vi "getDeviceType.vi"(8 "error in":errorcluster, 11 "connection ID":i32) -> (0 "error out":errorcluster, 2 "devicetype":string, 3 "connection ID":i32)   [LabVIEW 2016]
doc: "This function gets the device type based on its EEPROM configuration."
panel:
  out "params_cluster":cluster{"Numeric":i32}
  in  "Params_cluster":cluster{"Numeric":dbl}
  in  "results_cluster":cluster{"errNo":i32, "devicetype":string}
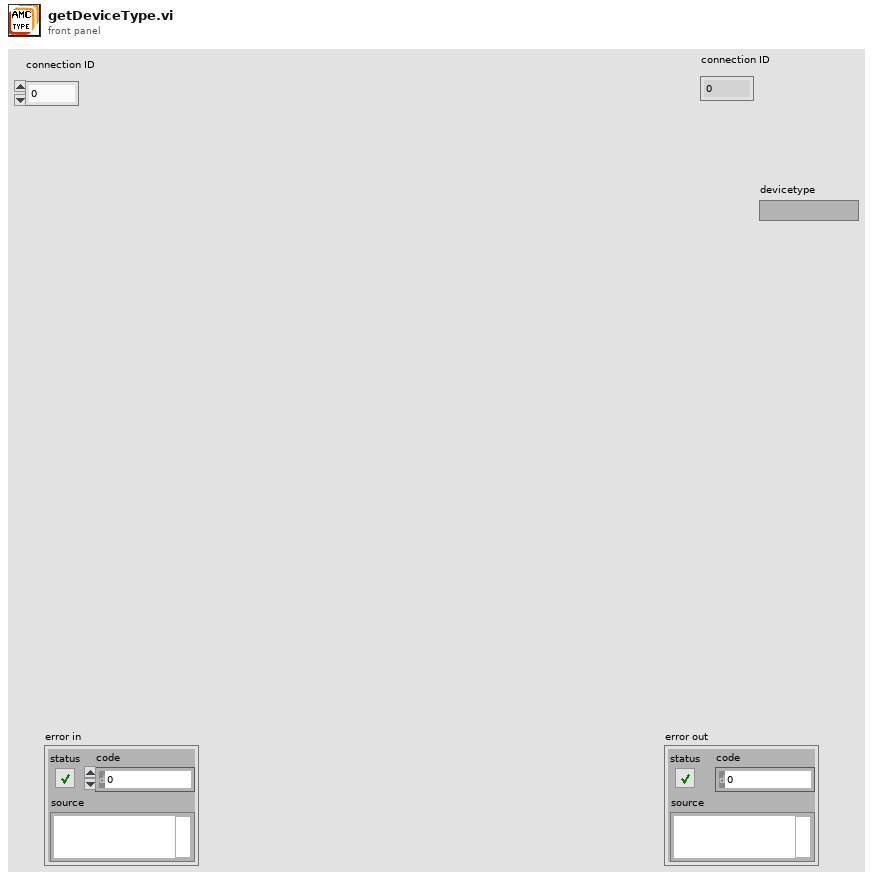
[diagram p1: front panel]
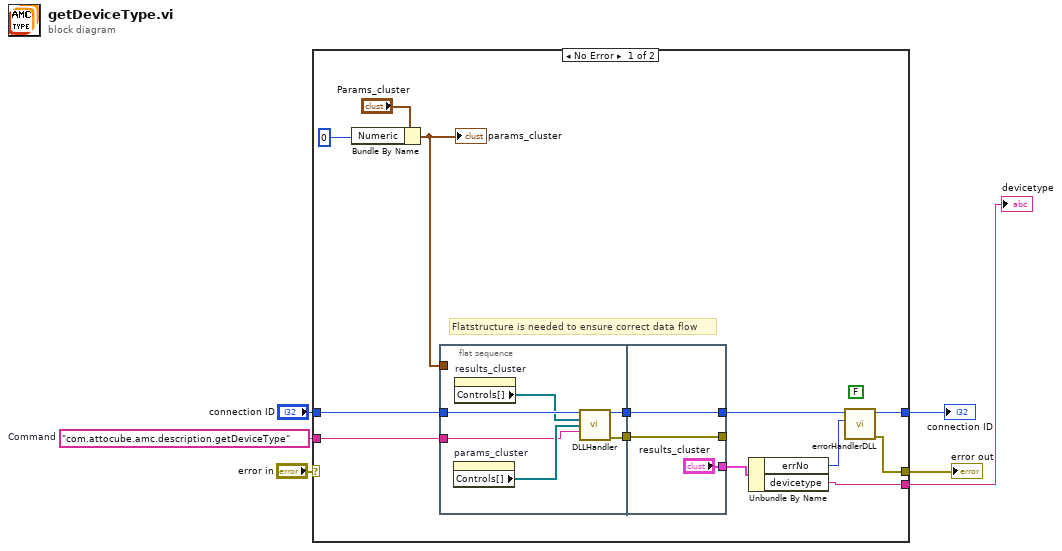
[diagram p0: block diagram]
diagram:
  w4 = "com.attocube.amc.description.getDeviceType"  # Command
  n1 = case shown="No Error" "error in" {
    selector: "error in" -> [_ w30]
    tunnel: [w9 w30] -> w6
    tunnel: "connection ID" -> [w19 w29]
    tunnel: w4 -> [w16 _]
    tunnel: [w11 w29] -> w2
    tunnel: [w7 _] -> w1
    frame No Error {
      (unwired) FALSE ("show popup")
      # "Flatstructure is needed to ensure correct data flow"
      n2 = Bundle By Name(cluster="Params_cluster", "Numeric"=0) -> (w14:cluster{"Numeric":dbl})
      "params_cluster" <- w14
      n3 = flat-sequence {
        tunnel: w19 -> [w25]
        tunnel: w16 -> [w22]
        tunnel: [w21] -> w15
        tunnel: w14 -> [_]
        tunnel: [w20] -> w12
        tunnel: ["results_cluster"] -> w18
        tunnel: [w28] -> w13
        tunnel: [w26] -> _
        tunnel: w15 -> [w26]
        tunnel: w12 -> [w28]
        frame #0 {
          n4 = property on="params_cluster" class="Clust (strict)"() -> ("Controls[]"=w23:refnum<vi>[])  [unwired: 2 in, 2 out]
          n5 = property on="results_cluster" class="Clust (strict)"() -> ("Controls[]"=w24:refnum<vi>[])  [unwired: 2 in, 2 out]
          n6 = call "DLLHandler.vi"("connection ID"=w25, "results_cluster"=w24, "params_cluster"=w23, "method"=w22) -> ("connection ID out"=w20:i32, "error"=w21:errorcluster)  [unwired: 10 in]
        }
        frame #1 {
        }
      }
      n7 = Unbundle By Name(w18) -> ("errNo"=w10:i32, "devicetype"=w7:string)
      n8 = call "errorHandlerDLL.vi"("error number"=w10, "connection ID"=w13) -> ("error out"=w9:errorcluster, "connection ID"=w11:i32)  [unwired: 8 in]
    }
    frame Error {
    }
  }
  "error out" <- w6
  "connection ID" <- w2
  "devicetype" <- w1
